vi "Extract Position Orientation Multi Tool.vi"(8 "Error In":errorcluster, 11 "Rigid Body Data":T4[](array[typedef])) -> (0 "Error Out":errorcluster, 3 "Rigid Bodies":T1[](array[typedef]))   [LabVIEW 2017]
uses:
  Controls/Raw Rigid Body Data.ctl
  Controls/Rigid Body Info.ctl
  Controls/Position.ctl
  Controls/Orientation.ctl
  <vilib>/Analysis/_algsub.llb/Vector Norm.vi
  <vilib>/Analysis/_algsub.llb/Real Vector Norm.vi
  <vilib>/Analysis/baseanly.llb/Outer Product.vi
  <vilib>/Analysis/baseanly.llb/Real Outer Product.vi
  <vilib>/robotics/Kinematics/Create Lie Group Matrix.vi
  <vilib>/Analysis/Matrix/Numeric/Multiply/Multiply.vi
  <vilib>/Analysis/Matrix/Numeric/Multiply/Multiply - RM,R.vi
  <vilib>/Analysis/Matrix/Numeric/Multiply/Multiply - R,RM.vi
  <vilib>/Analysis/Matrix/Numeric/Add/Add.vi
  <vilib>/Analysis/Matrix/Numeric/Add/Add - RM,RM.vi
  <vilib>/robotics/Kinematics/NI_Kinematics.lvlib
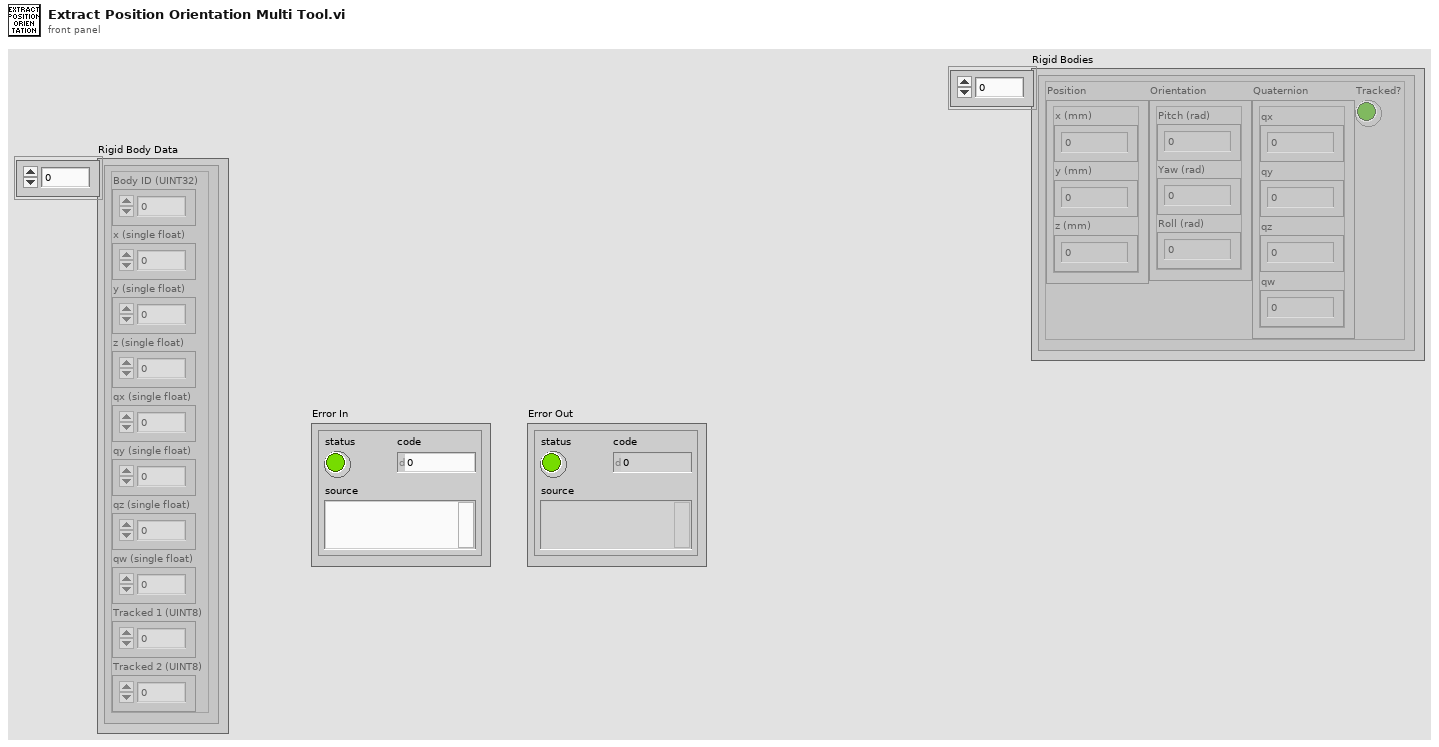
[diagram p1: front panel]
types:
  T1 = typedef "Rigid Body Info.ctl" = cluster{"Position":T2, "Orientation":T3, "Quaternion":cluster{"qx":sgl, "qy":sgl, "qz":sgl, "qw":sgl}, "Tracked?":bool}
  T2 = typedef "Position.ctl" = cluster{"x (mm)":sgl, "y (mm)":sgl, "z (mm)":sgl}
  T3 = typedef "Orientation.ctl" = cluster{"Pitch (rad)":sgl, "Yaw (rad)":sgl, "Roll (rad)":sgl}
  T4 = typedef "Raw Rigid Body Data.ctl" = cluster{"Body ID (UINT32)":u32, "x (single float)":sgl, "y (single float)":sgl, "z (single float)":sgl, "qx (single float)":sgl, "qy (single float)":sgl, "qz (single float)":sgl, "qw (single float)":sgl, "Tracked 1 (UINT8)":u8, "Tracked 2 (UINT8)":u8}
  T5 = typedef "NI_Kinematics.lvlib/Quaternion.ctl" = dbl[]
  T6 = typedef "NI_Matrix.lvlib/RealMatrix.ctl" = dbl[][]
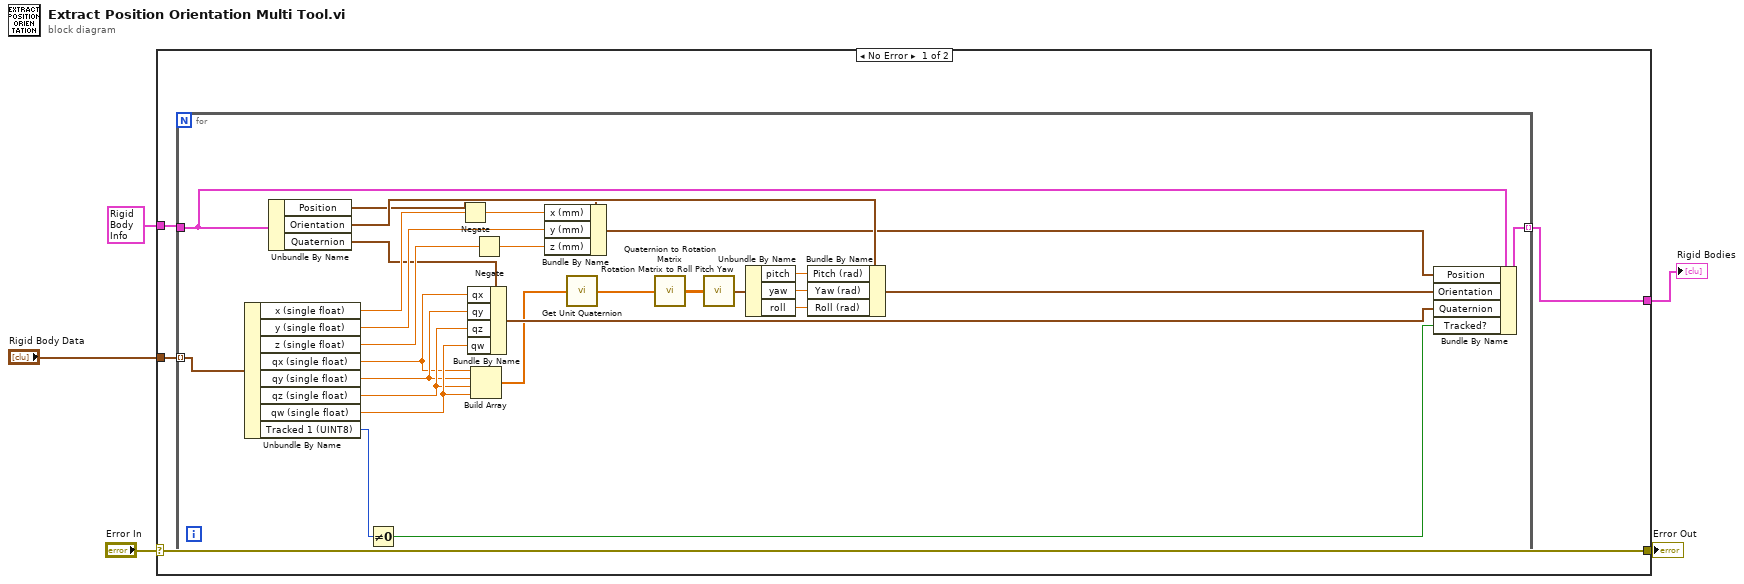
[diagram p0: block diagram]
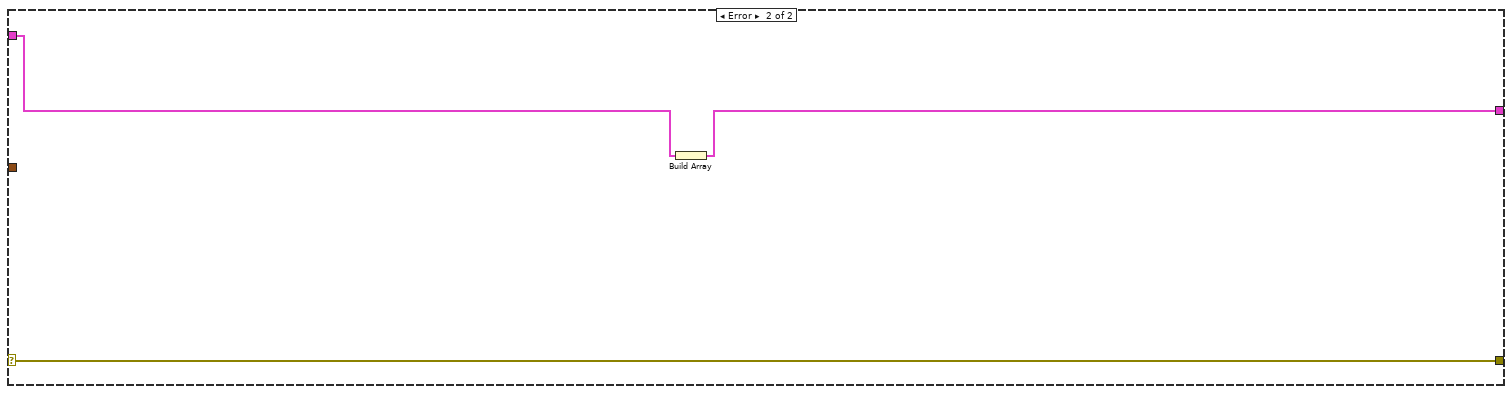
[diagram p2: hidden frame]
diagram:
  n1 = case shown="No Error" "Error In" {
    selector: "Error In" -> [w7 w39]
    tunnel: [w9 w37] -> w1
    tunnel: T1 {"Position"={"x (mm)"=0.0, "y (mm)"=0.0, "z (mm)"=0.0}, "Orientation"={"Pitch (rad)"=-180.0, "Yaw (rad)"=-0.0, "Roll (rad)"=-180.0}, "Quaternion"={"qx"=0.0, "qy"=0.0, "qz"=0.0, "qw"=0.0}, "Tracked?"=FALSE} ("Rigid Body") -> [w8 w38]
    tunnel: "Rigid Body Data" -> [w6 _]
    tunnel: [w7 w39] -> w2
    frame No Error {
      n2 = for {
        tunnel: w6 -> [w10] mode=indexing
        tunnel: w8 -> [w34]
        tunnel: [w36] -> w9 mode=indexing
        n3 = Unbundle By Name(w10) -> ("x (single float)"=w28:sgl, "y (single float)"=w27:sgl, "z (single float)"=w26:sgl, "qx (single float)"=w30:sgl, "qy (single float)"=w31:sgl, "qz (single float)"=w32:sgl, "qw (single float)"=w33:sgl, "Tracked 1 (UINT8)"=w29:u8)
        n4 = Unbundle By Name(w34) -> ("Position"=w23:T2, "Orientation"=w25:T3, "Quaternion"=w21:cluster{"qx":sgl, "qy":sgl, "qz":sgl, "qw":sgl})
        n5 = Not Equal To 0?(x=w29) -> (x != 0?=w35:bool)
        n6 = Negate(x=w28) -> (-x=w11:sgl)
        n7 = Bundle By Name(cluster=w21, "qx"=w30, "qy"=w31, "qz"=w32, "qw"=w33) -> (w20:cluster{"qx":sgl, "qy":sgl, "qz":sgl, "qw":sgl})
        n8 = Build Array(w30, w31, w32, w33) -> (w13:sgl[])
        n9 = Negate(x=w26) -> (-x=w14:sgl)
        n10 = Bundle By Name(cluster=w23, "x (mm)"=w11, "y (mm)"=w27, "z (mm)"=w14) -> (w22:T2)
        n11 = call <vilib>:"Get Unit Quaternion.vi"("quaternion"=w13) -> ("unit quaternion"=w12:T5)
        n12 = call <vilib>:"Quaternion to Rotation Matrix.vi"("quaternion"=w12) -> ("rotation matrix"=w18:T6)
        n13 = call <vilib>:"Rotation Matrix to Roll Pitch Yaw.vi"("rotation matrix"=w18) -> ("angles"=w19:cluster{"roll":dbl, "pitch":dbl, "yaw":dbl})
        n14 = Unbundle By Name(w19) -> ("pitch"=w15:dbl, "yaw"=w16:dbl, "roll"=w17:dbl)
        n15 = Bundle By Name(cluster=w25, "Pitch (rad)"=w15, "Yaw (rad)"=w16, "Roll (rad)"=w17) -> (w24:T3)
        n16 = Bundle By Name(cluster=w34, "Position"=w22, "Orientation"=w24, "Quaternion"=w20, "Tracked?"=w35) -> (w36:T1)
      }
    }
    frame Error {
      n17 = Build Array(w38) -> (w37:T1[])
    }
  }
  "Error Out" <- w2
  "Rigid Bodies" <- w1
